vi "SW_Load_proc_data_from_TDMS.vi"(8 "error in (no error)":errorcluster, 11 "TDMS track ref. in":path) -> (0 "error out":errorcluster, 2 "Rec start Time Stamp":timestamp, 3 "Loaded data output":T1)   [LabVIEW 2018, in "Tracker.lvlib"]
uses:
  Tracker.lvlib
  Controls/CTL_Loaded_data_output_(offline).ctl
  Common_Resources.lvlib
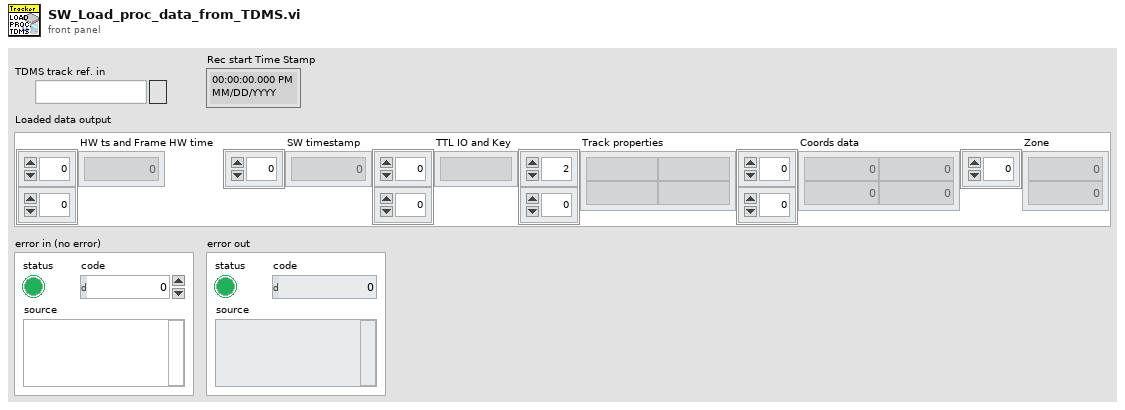
[diagram p1: front panel]
types:
  T1 = typedef "Common_Resources.lvlib/CTL_Loaded_data_output_(offline).ctl" = cluster{"HW ts and Frame HW time":u32[][], "SW timestamp":dbl[], "TTL IO and Key":string[][], "Track properties":string[][], "Coords data":dbl[][], "Zone":i8[]}
  T2 = enum16{"big-endian, network order", "native, host order", "little-endian"}
  T3 = enum16{"open", "open or create", "create or replace", "create", "open (read-only)"}
  T4 = cluster{"Absolute timestamp (DBL)":dbl[], "Relative timestamp (DBL)":dbl[], "Zones normalized allocation array":dbl[][], "Coordinates and speed":dbl[][], "Current zone and TTLs":u8[][], "Acquisition settings cluster out":cluster{"Researcher name":string, "N segments MIDFIELD":u8, "N segments BORDER":u8, "Radius, mm CENTER":u16, "Radius, mm MIDFIELD":u16, "Starting angle MIDFIELD":i16, "Starting angle BORDER":i16, "Cage diameter, mm":u16, "Bridge swap":bool, "Bridge V. offset":sgl, "Twisted neck":bool, "Offset H.":sgl, "Name prefix":string, "Stop at":dbl, "\"Stop at\" enabled":bool, "Settings loaded OK":bool}, "Stimulus presets array":cluster{"Event type":u16, "Time, s":sgl, "Stimulus, s":sgl, "Set/Clear":bool, "TTL out":u16, "Stim. has been set":bool}[]}
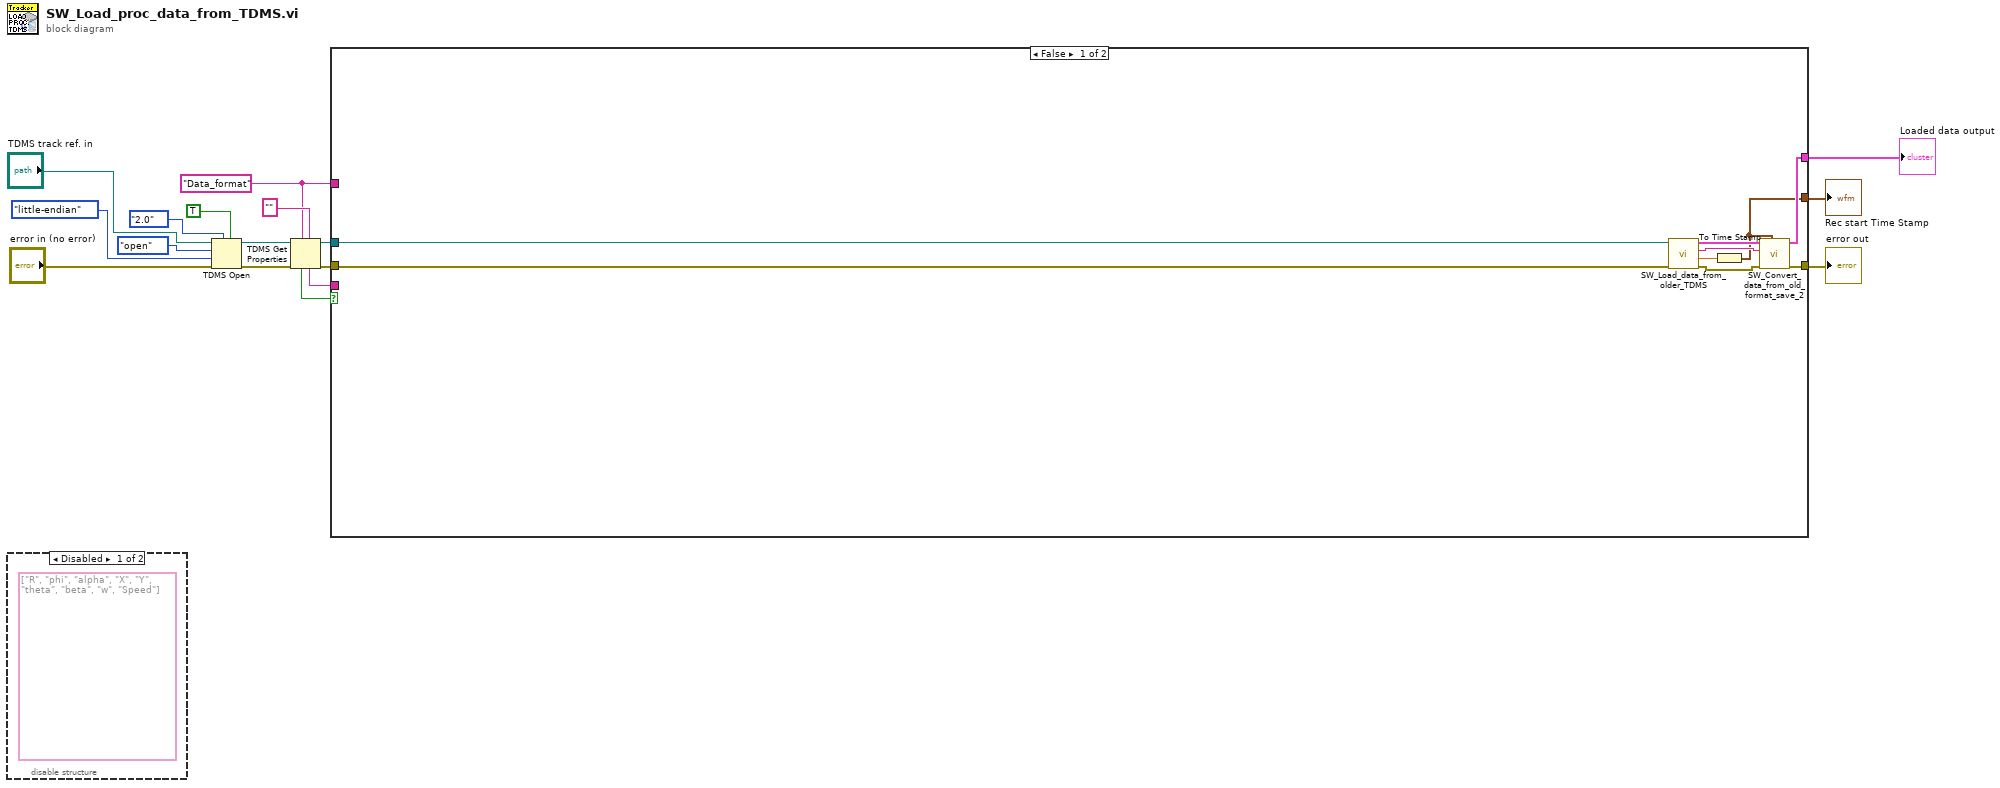
[diagram p0: block diagram]
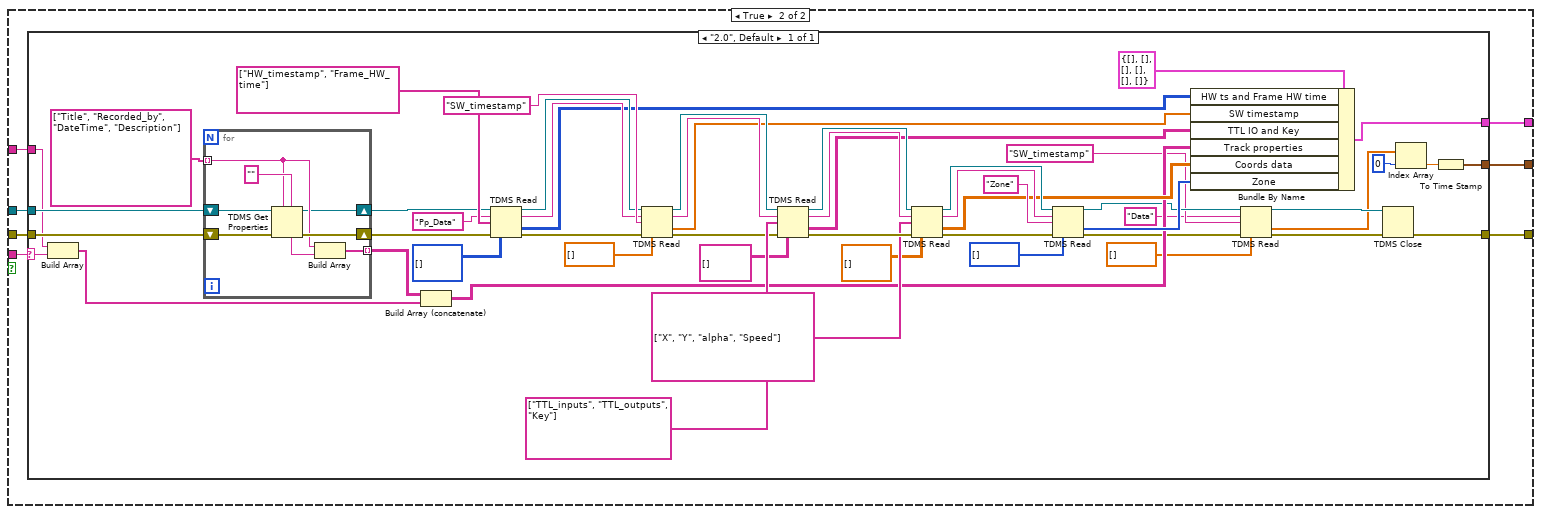
[diagram p2: hidden frame]
diagram:
  w2 = "Data_format"
  n1 = disable-structure shown="Disabled" {
    frame Disabled {
      (unwired) string[] ["R", "phi", "alpha", "X", "Y", "theta", "beta", "w", "Speed"] ("appended array")
    }
    frame Enabled {
    }
  }
  n2 = TDMS Open(5:TRUE ("create index file? (T)"), 7:enum16{"1.0", "2.0"}."2.0" ("file format version (2.0)"), 8:"error in (no error)", 9:T2."little-endian" ("byte order (2:little-endian)"), 10:T3."open" ("operation (0:open)"), 11:"TDMS track ref. in") -> (0:w9:errorcluster, 3:w10:refnum<k34>)  [unwired: 1 in]
  n3 = TDMS Get Properties(5:"", 7:w2, 8:w9, 11:w10) -> (0:w8:errorcluster, 3:w7:refnum<k34>, 4:w5:string, 6:w6:bool)  [unwired: 2 in, 2 out]
  n4 = case shown="False" w6 {
    tunnel: w8 -> [w26 w33]
    tunnel: w7 -> [w25 w32]
    tunnel: w5 -> [_ w31]
    tunnel: [w21 w30] -> w4
    tunnel: [w20 w29] -> w3
    tunnel: w2 -> [_ w28]
    tunnel: [w18 w27] -> w1
    frame False {
      n5 = call "SW_Load_data_from_older_TDMS.vi"("error in (no error)"=w26, "TDMS file ref."=w25) -> ("error out"=w23:errorcluster, "Start time"=w19:dbl, "Author's name"=w22:string, "Loaded data"=w24:T4)  [unwired: 4 in, 2 out]
      n6 = To Time Stamp(1:w19) -> (0:w18:timestamp)
      n7 = call "SW_Convert_data_from_old_format_save_2.vi"("Time Stamp in"=w18, "error in (no error)"=w23, "Researcher name"=w22, "Loaded data in"=w24) -> ("error out"=w20:errorcluster, "Loaded data out"=w21:T1)  [unwired: 6 in]
    }
    frame True {
      n8 = case shown="\"2.0\", Default" w31 {
        selector: w31 -> [w49]
        tunnel: w33 -> [w52]
        tunnel: w32 -> [w51]
        tunnel: [w47] -> w30
        tunnel: [w46] -> w29
        tunnel: w28 -> [w45]
        tunnel: [w34] -> w27
        frame "2.0", Default {
          n9 = Build Array(w45, w49) -> (w48:string[])
          n10 = for {
            tunnel: string[] ["Title", "Recorded_by", "DateTime", "Description"] ("property names") -> [w89] mode=indexing
            tunnel: [w87] -> w54 mode=indexing
            shift-right: [w86] -> w70
            shift-left: w51 -> [w92]
            shift-right: [w90] -> w71
            shift-left: w52 -> [w93]
            n11 = TDMS Get Properties(5:"", 7:w89, 8:w93, 11:w92) -> (0:w90:errorcluster, 3:w86:refnum<k34>, 4:w88:string)  [unwired: 2 in, 3 out]
            n12 = Build Array(w89, w88) -> (w87:string[])
          }
          n13 = Build Array (concatenate)(w54, w48) -> (w50:string[][])
          n14 = TDMS Read(0:w70, 5:"Pp_Data" ("group name in"), 7:string[] ["HW_timestamp", "Frame_HW_time"] ("appended array"), 11:w71, 12:u32[][] [] ("appended array")) -> (4:w77:refnum<k34>, 6:w76:string, 10:w58:u32[][], 15:w75:errorcluster)  [unwired: 3 in, 2 out]
          n15 = TDMS Read(0:w77, 5:w76, 7:"SW_timestamp" ("channel name(s) in (Untitled)"), 11:w75, 12:dbl[] [] ("appended array")) -> (4:w80:refnum<k34>, 6:w82:string, 10:w57:dbl[], 15:w81:errorcluster)  [unwired: 3 in, 2 out]
          n16 = TDMS Read(0:w80, 5:w82, 7:string[] ["TTL_inputs", "TTL_outputs", "Key"] ("channel name(s) in (Untitled)"), 11:w81, 12:string[][] [] ("appended array")) -> (4:w69:refnum<k34>, 6:w68:string, 10:w53:string[][], 15:w67:errorcluster)  [unwired: 3 in, 2 out]
          n17 = TDMS Read(0:w69, 5:w68, 7:string[] ["X", "Y", "alpha", "Speed"] ("appended array"), 11:w67, 12:dbl[][] [] ("appended array")) -> (4:w63:refnum<k34>, 6:w62:string, 10:w56:dbl[][], 15:w64:errorcluster)  [unwired: 3 in, 2 out]
          n18 = TDMS Read(0:w63, 5:w62, 7:"Zone", 11:w64, 12:i8[] [] ("appended array")) -> (4:w43:refnum<k34>, 10:w55:i8[], 15:w44:errorcluster)  [unwired: 3 in, 3 out]
          n19 = Bundle By Name(cluster=T1 {"HW ts and Frame HW time"=[], "SW timestamp"=[], "TTL IO and Key"=[], "Track properties"=[], "Coords data"=[], "Zone"=[]} ("Loaded data output"), "HW ts and Frame HW time"=w58, "SW timestamp"=w57, "TTL IO and Key"=w53, "Track properties"=w50, "Coords data"=w56, "Zone"=w55) -> (w47:T1)
          n20 = TDMS Read(0:w43, 5:"Data" ("group name in"), 7:"SW_timestamp" ("channel name(s) in (Untitled)"), 11:w44, 12:dbl[] [] ("appended array")) -> (4:w42:refnum<k34>, 10:w37:dbl[], 15:w41:errorcluster)  [unwired: 3 in, 3 out]
          n21 = TDMS Close(8:w41, 11:w42) -> (0:w46:errorcluster)  [unwired: 1 out]
          n22 = Index Array(array=w37, index=0) -> (element=w35:dbl)
          n23 = To Time Stamp(1:w35) -> (0:w34:timestamp)
        }
      }
    }
  }
  "Loaded data output" <- w4
  "error out" <- w3
  "Rec start Time Stamp" <- w1
